vi "QueryDetermineLayer.vi"(8 "error in (no error)":errorcluster, 10 "Query":T1, 11 "FAMM in":refnum<class "FAMM.lvclass">) -> (0 "error out":errorcluster, 2 "Memory_Layer":i32, 3 "FAMM out":refnum<class "FAMM.lvclass">)   [LabVIEW 2020, in "FAMM.lvclass"]
doc: "Determine on which memory layer to perform the request"
uses:
  FAMM.lvclass
  controls/FAMMrequest.ctl
  Gview/controls/Typedef_Live.ctl
  FAMM.lvclass/FAMM.ctl
  Gview/Gviewer.lvclass
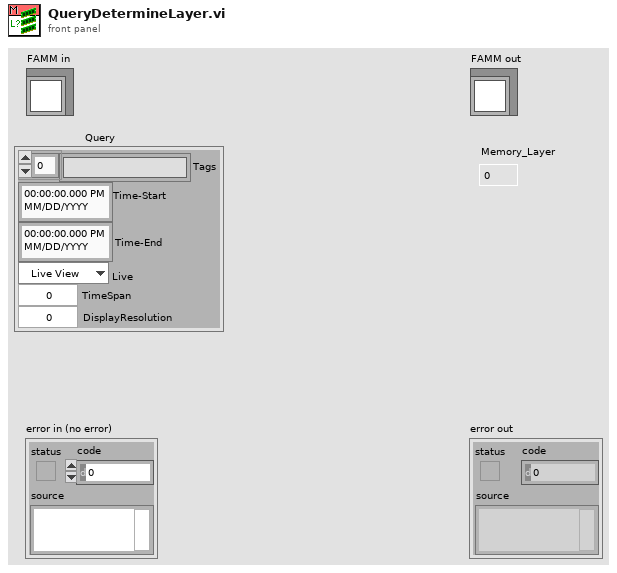
[diagram p1: front panel]
types:
  T1 = typedef "FAMM.lvclass/FAMMrequest.ctl" = cluster{"Tags":string[], "Time-Start":timestamp, "Time-End":timestamp, "Live":T2, "TimeSpan":dbl, "DisplayResolution":i32}
  T2 = typedef "Gviewer.lvclass/Typedef_Live.ctl" = enum16{"Live View", "Freeze"}
  T3 = typedef "FAMM.lvclass/FAMM-attributes.ctl" = cluster{"FAMM_PAQ_Layers":i32, "FAMM_PAQ_resolution":dbl, "PAQ_TAGs":string[], "WAQ_TAGs":string[], "EAQ_TAGs":string[], "All_TAGs":string[], "PAQtagProps":T4[], "WAQtagProps":T4[], "EAQtagProps":T4[], "DBAL_class":refnum<data-value>, "PAQ_memory":refnum<data-value>[], "PAQupdates":timestamp[], "FAMM_Size":cluster{"other":i32, "1day":i32, "1week":i32}, "DatabaseFileExtention":string, "DatabaseSaveRate":dbl, "Database_path":path, "DBAL-Queue":refnum<queue>}
  T4 = typedef "typedef_com_TagProp.ctl" = cluster{"Description":string, "EngUnits":string, "RangeH":dbl, "RangeL":dbl, "Resolution":i32, "Obsolete":bool, "ChangeDate":timestamp, "ChangeSource":string, "ChangeReason":string, "TagFunc":u32}
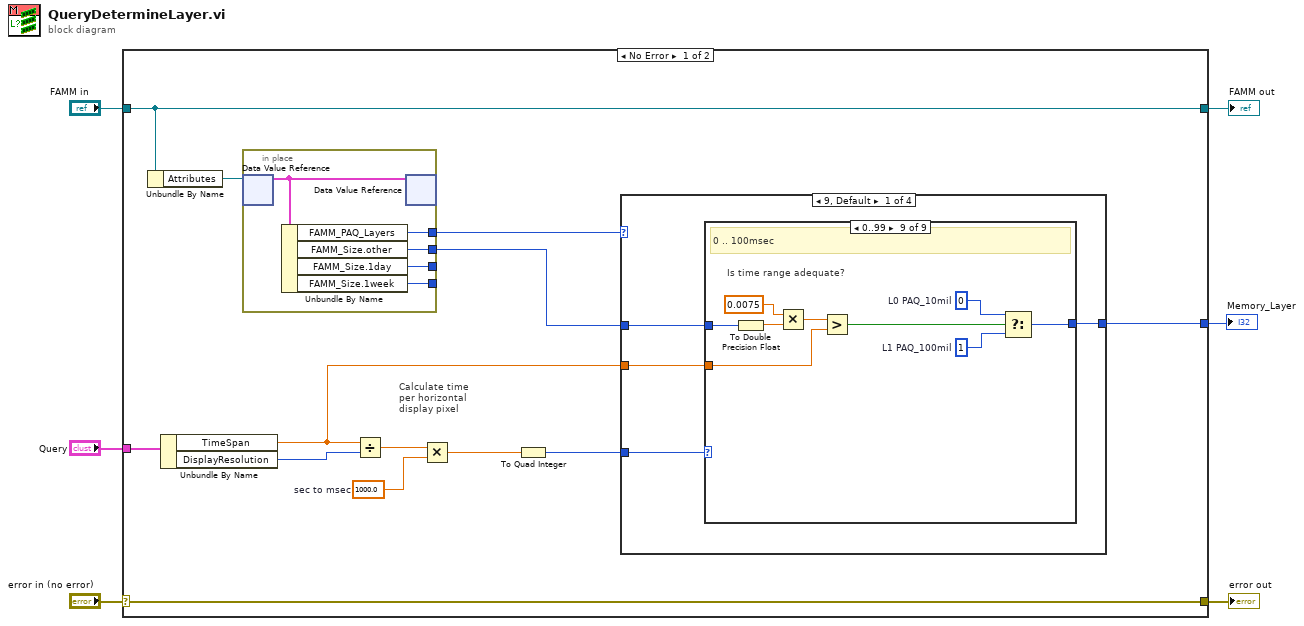
[diagram p0: block diagram]
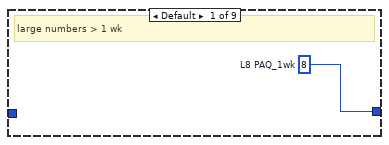
[diagram p2: hidden frame]
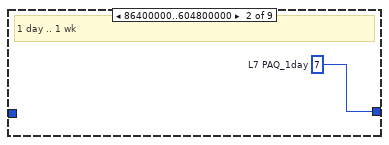
[diagram p3: hidden frame]
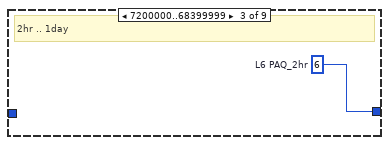
[diagram p4: hidden frame]
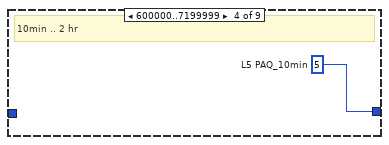
[diagram p5: hidden frame]
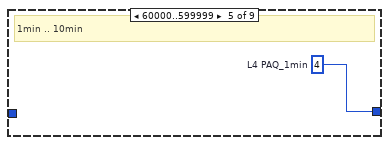
[diagram p6: hidden frame]
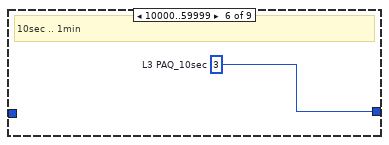
[diagram p7: hidden frame]
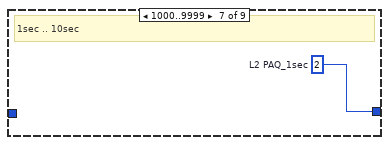
[diagram p8: hidden frame]
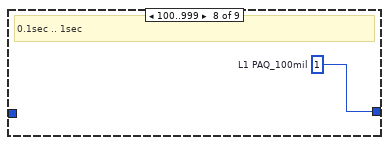
[diagram p9: hidden frame]
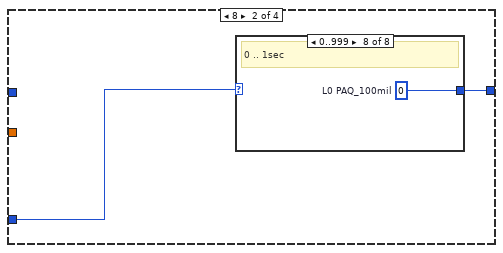
[diagram p10: hidden frame]
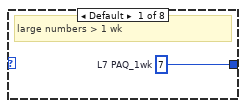
[diagram p11: hidden frame]
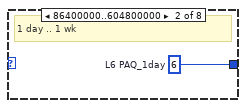
[diagram p12: hidden frame]
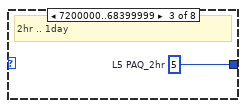
[diagram p13: hidden frame]
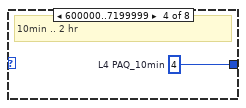
[diagram p14: hidden frame]
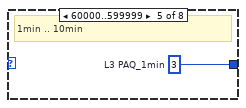
[diagram p15: hidden frame]
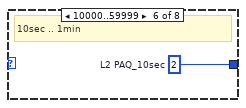
[diagram p16: hidden frame]
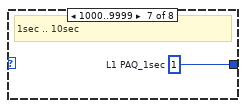
[diagram p17: hidden frame]
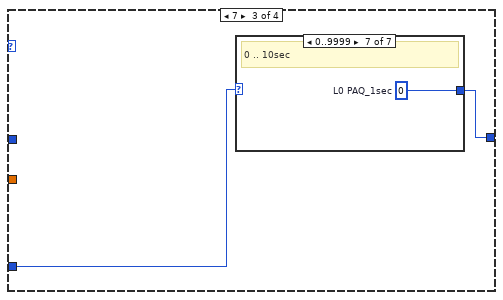
[diagram p18: hidden frame]
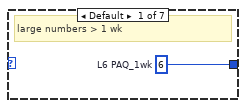
[diagram p19: hidden frame]
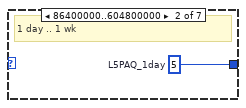
[diagram p20: hidden frame]
diagram:
  n1 = case shown="No Error" "error in (no error)" {
    selector: "error in (no error)" -> [w19 w75]
    tunnel: [w19 w75] -> w5
    tunnel: [w18 w74] -> w3
    tunnel: "FAMM in" -> [w18 w74]
    tunnel: "Query" -> [w10 _]
    tunnel: [w9 -1 ("L0 PAQ_10sec")] -> w1
    frame No Error {
      w12 = 1000.0  # sec to msec
      # "Calculate time\nper horizontal\ndisplay pixel"
      n2 = Unbundle By Name(w18) -> ("Attributes"=w17:refnum<data-value>)
      n3 = Unbundle By Name(w10) -> ("TimeSpan"=w7:dbl, "DisplayResolution"=w13:i32)
      n4 = in-place {
        in-place-border: [w71] -> w11
        in-place-border: [w70] -> w8
        in-place-border: [w69] -> _
        in-place-border: [w68] -> _
        n5 = in-place-dvr #1(w17) -> (w72:T3)  [unwired: 1 out]
        n6 = Unbundle By Name(w72) -> ("FAMM_PAQ_Layers"=w71:i32, "FAMM_Size.other"=w70:i32, "FAMM_Size.1day"=w69:i32, "FAMM_Size.1week"=w68:i32)
        n7 = in-place-dvr #1(w72) -> ()  [unwired: 2 out]
      }
      n8 = Divide(x=w7, y=w13) -> (x/y=w14:dbl)
      n9 = Multiply(x=w14, y=w12) -> (x*y=w15:dbl)
      n10 = To Quad Integer(1:w15) -> (0:w16:i64)
      n11 = case shown="9, Default" w11 {
        tunnel: w16 -> [w23 w42 w52 w61]
        tunnel: [w22 w41 w51 w60] -> w9
        tunnel: w8 -> [w21 _ _ _]
        tunnel: w7 -> [w20 _ _ _]
        frame 9, Default {
          n12 = case shown="0..99" w23 {
            tunnel: [w24 w25 w26 w27 w28 w29 w30 w31 w32] -> w22
            tunnel: w21 -> [_ _ _ _ _ _ _ _ w40]
            tunnel: w20 -> [_ _ _ _ _ _ _ _ w36]
            frame Default {
              w24 = 8  # L8 PAQ_1wk
              # "large numbers > 1 wk"
            }
            frame 86400000..604800000 {
              w25 = 7  # L7 PAQ_1day
              # "1 day .. 1 wk"
            }
            frame 7200000..68399999 {
              w26 = 6  # L6 PAQ_2hr
              # "2hr .. 1day"
            }
            frame 600000..7199999 {
              w27 = 5  # L5 PAQ_10min
              # "10min .. 2 hr"
            }
            frame 60000..599999 {
              w28 = 4  # L4 PAQ_1min
              # "1min .. 10min"
            }
            frame 10000..59999 {
              w29 = 3  # L3 PAQ_10sec
              # "10sec .. 1min"
            }
            frame 1000..9999 {
              w30 = 2  # L2 PAQ_1sec
              # "1sec .. 10sec"
            }
            frame 100..999 {
              w31 = 1  # L1 PAQ_100mil
              # "0.1sec .. 1sec"
            }
            frame 0..99 {
              w33 = 1  # L1 PAQ_100mil
              w34 = 0  # L0 PAQ_10mil
              # "Is time range adequate?"
              # "0 .. 100msec"
              n13 = To Double Precision Float(number=w40) -> (double precision float=w39:dbl)
              n14 = Multiply(x=0.0075, y=w39) -> (x*y=w37:dbl)
              n15 = Greater?(x=w37, y=w36) -> (0:w35:bool)
              n16 = Select(t=w34, s=w35, f=w33) -> (s? t:f=w32:i32)
            }
          }
        }
        frame 8 {
          n17 = case shown="0..999" w42 {
            tunnel: [w43 w44 w45 w46 w47 w48 w49 w50] -> w41
            frame Default {
              w43 = 7  # L7 PAQ_1wk
              # "large numbers > 1 wk"
            }
            frame 86400000..604800000 {
              w44 = 6  # L6 PAQ_1day
              # "1 day .. 1 wk"
            }
            frame 7200000..68399999 {
              w45 = 5  # L5 PAQ_2hr
              # "2hr .. 1day"
            }
            frame 600000..7199999 {
              w46 = 4  # L4 PAQ_10min
              # "10min .. 2 hr"
            }
            frame 60000..599999 {
              w47 = 3  # L3 PAQ_1min
              # "1min .. 10min"
            }
            frame 10000..59999 {
              w48 = 2  # L2 PAQ_10sec
              # "10sec .. 1min"
            }
            frame 1000..9999 {
              w49 = 1  # L1 PAQ_1sec
              # "1sec .. 10sec"
            }
            frame 0..999 {
              w50 = 0  # L0 PAQ_100mil
              # "0 .. 1sec"
            }
          }
        }
        frame 7 {
          n18 = case shown="0..9999" w52 {
            tunnel: [w53 w54 w55 w56 w57 w58 w59] -> w51
            frame Default {
              w53 = 6  # L6 PAQ_1wk
              # "large numbers > 1 wk"
            }
            frame 86400000..604800000 {
              w54 = 5  # L5PAQ_1day
              # "1 day .. 1 wk"
            }
            frame 7200000..68399999 {
              w55 = 4  # L4 PAQ_2hr
              # "2hr .. 1day"
            }
            frame 600000..7199999 {
              w56 = 3  # L3 PAQ_10min
              # "10min .. 2 hr"
            }
            frame 60000..599999 {
              w57 = 2  # L2 PAQ_1min
              # "1min .. 10min"
            }
            frame 10000..59999 {
              w58 = 1  # L1 PAQ_10sec
              # "10sec .. 1min"
            }
            frame 0..9999 {
              w59 = 0  # L0 PAQ_1sec
              # "0 .. 10sec"
            }
          }
        }
        frame 6 {
          n19 = case shown="Default" w61 {
            tunnel: [w62 w63 w64 w65 w66 w67] -> w60
            frame Default {
              w62 = 5  # L5 PAQ_1wk
              # "large numbers > 1 wk"
            }
            frame 86400000..604800000 {
              w63 = 4  # L4PAQ_1day
              # "1 day .. 1 wk"
            }
            frame 7200000..68399999 {
              w64 = 3  # L3 PAQ_2hr
              # "2hr .. 1day"
            }
            frame 600000..7199999 {
              w65 = 2  # L2 PAQ_10min
              # "10min .. 2 hr"
            }
            frame 60000..599999 {
              w66 = 1  # L1 PAQ_1min
              # "1min .. 10min"
            }
            frame 0..59999 {
              w67 = 0  # L0 PAQ_10sec
              # "10sec .. 1min"
            }
          }
        }
      }
    }
    frame Error {
    }
  }
  "error out" <- w5
  "FAMM out" <- w3
  "Memory_Layer" <- w1
